vi "Read Log Lines.vi"(8 "error in (no error)":errorcluster, 11 "filePath":path) -> (0 "error out":errorcluster, 3 "lines":string[](array[string]))   [LabVIEW 2026, in "Tests.lvlib"]
doc: "Test readback helper for file-mechanics tests. Recursively lists log files under a root folder matching the given extension, returned sorted by path, so tests can assert how many files were written and where (including calendar sub-folders created when calendarFolderTree is enabled). Call only after Shutdown has flushed and closed the files, the appender holds the current file open until CloseSink. Pure read; does not modify the tree."
uses:
  Tests.lvlib
  <vilib>/Utility/error.llb/Trim Whitespace (string).vi
  <vilib>/Utility/error.llb/Trim Whitespace One-Sided.vi
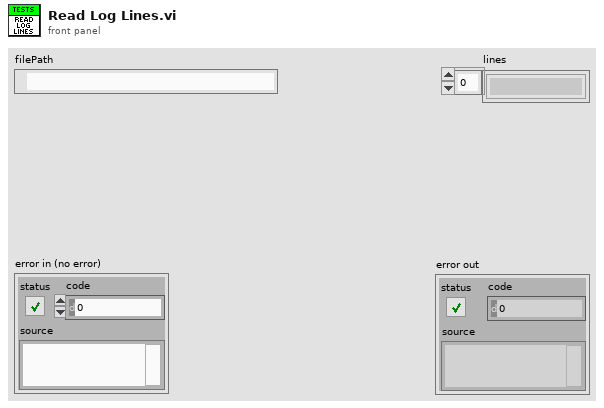
[diagram p1: front panel]
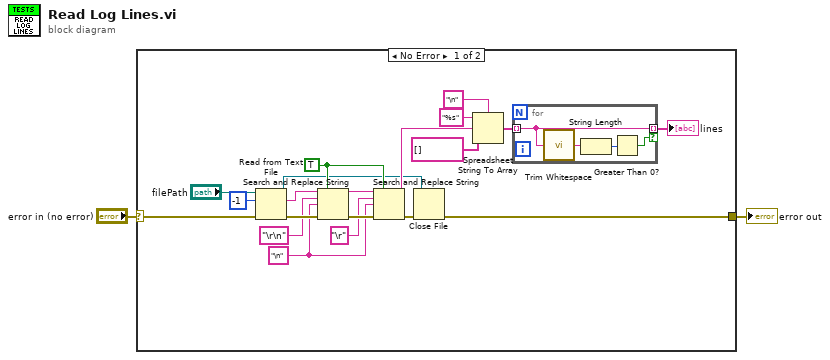
[diagram p0: block diagram]
diagram:
  n1 = case shown="No Error" "error in (no error)" {
    selector: "error in (no error)" -> [w22 w27]
    tunnel: [w4 w27] -> w2
    frame No Error {
      w13 = "\n" ("search string")
      w16 = TRUE ("replace all? (F)")
      n2 = Read from Text File(file (use dialog)="filePath", count=-1, error in=w22) -> (refnum out=w3:refnum<file>, text=w18:string, error out=w19:errorcluster)  [unwired: 1 in, 1 out]
      n3 = Search and Replace String(replace all?=w16, input string=w18, search string="\r\n", replace string=w13, error in=w19) -> (result string=w12:string, error out=w17:errorcluster)  [unwired: 3 in, 2 out]
      n4 = Search and Replace String(replace all?=w16, input string=w12, search string="\r", replace string=w13, error in=w17) -> (result string=w11:string, error out=w5:errorcluster)  [unwired: 3 in, 2 out]
      n5 = Close File(refnum=w3, error in=w5) -> (error out=w4:errorcluster)  [unwired: 1 out]
      n6 = Spreadsheet String To Array(delimiter (Tab)="\n", format string="%s", spreadsheet string=w11, array type (2D Dbl)=string[] []) -> (array=w7:string[])
      n7 = for {
        tunnel: w7 -> [w26] mode=indexing
        tunnel: [w26] -> w6 mode=indexing if=w23
        n8 = call-poly <vilib>:"Trim Whitespace.vi"("string"=w26) -> ("trimmed string"=w25:string)  [unwired: 1 in]
        n9 = String Length(string=w25) -> (length=w24:i32)
        n10 = Greater Than 0?(x=w24) -> (x > 0?=w23:bool)
      }
      "lines" <- w6
    }
    frame Error {
    }
  }
  "error out" <- w2
